vi "Calculate_Tolerance.vi"(2 "error in (no error)":errorcluster, 3 "State":T1=enum."Wait for something", 4 "Data":T2 {"Shaft"."dmin" format="%#_7g"; "Shaft"."dmax" format="%#_7g"; "Shaft"."Fundamental Dev" format="%#_7g"; "Shaft"."Tolerance Grade (IT) Shaft" format="%#_7g"; "Hole"."Dmin" format="%#_7g"; "Hole"."Tolerance Grade (IT)" format="%#_7g"}) -> (0 "error out":errorcluster, 1 "State":T1=enum."Wait for something")   [LabVIEW 2023]
uses:
  TypeDef/Data_Cluster.ctl
  <vilib>/MGI/Panel Manager/Panel/Panel/Window/Window.lvclass
  TypeDef/Units.ctl
  TypeDef/Method_Info.ctl
  TypeDef/Hole_Data.ctl
  TypeDef/Shaft_Data.ctl
  TypeDef/State.ctl
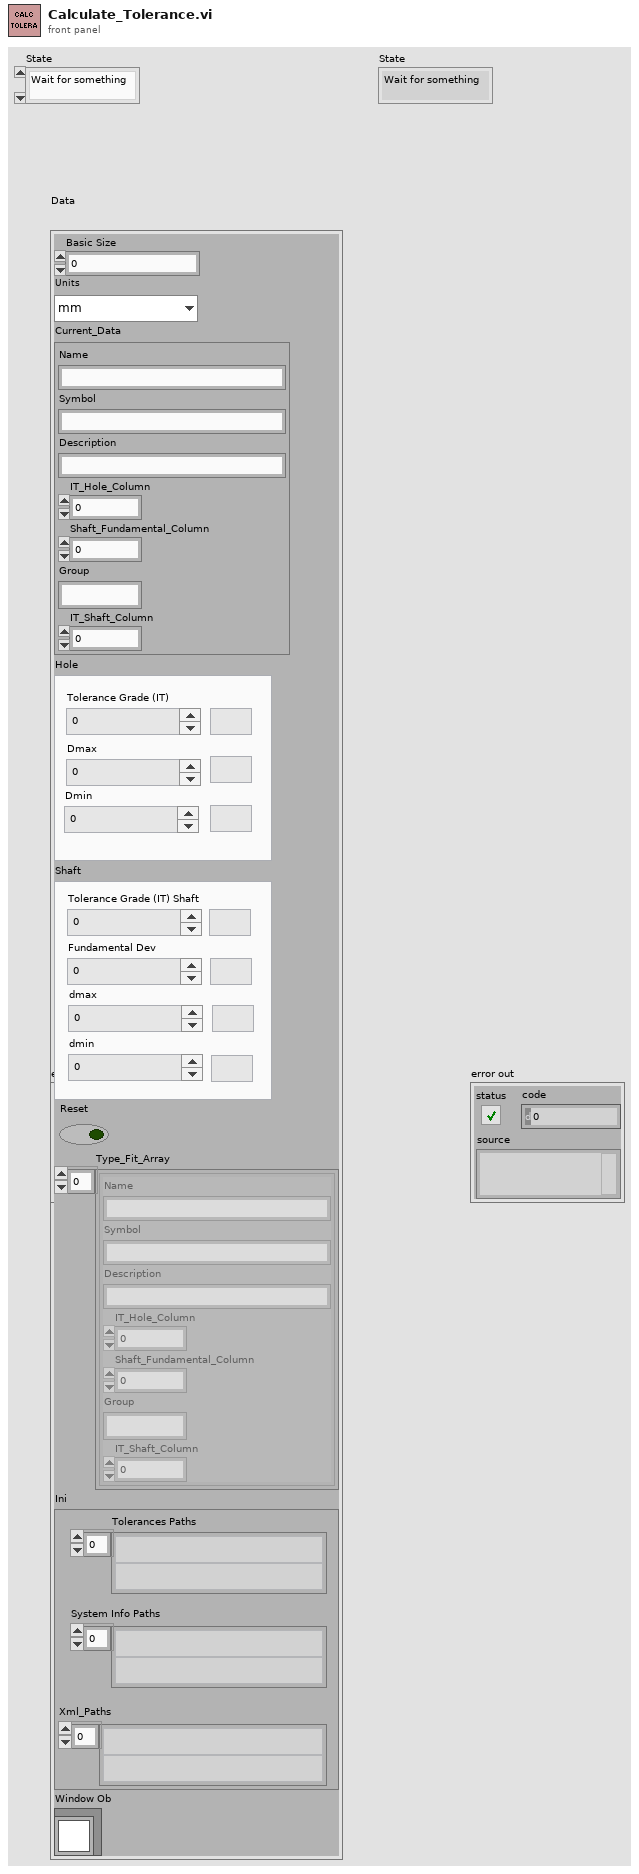
[diagram p1: front panel]
types:
  T1 = typedef "State.ctl" = enum16{"Initialize", "Wait for something", "Method_Description", "Tolerance Grade Hole", "Dmax-min", "Shaft Fudamental", "Shaft Tolerance Grade", "dmax-dmin", "Display Values"}
  T2 = typedef "Data_Cluster.ctl" = cluster{"Basic Size ":dbl, "Units":T3, "Current_Data":T4, "Hole":T5, "Shaft":T6, "Reset":bool, "Type_Fit_Array":T4[], "Ini":cluster{"Tolerances Paths":path[], "System Info Paths":path[], "Xml_Paths":path[]}, "Window Ob":refnum<class "Window.lvclass">}
  T3 = typedef "Units.ctl" = enum16{"mm", "in"}
  T4 = typedef "Method_Info.ctl" = cluster{"Name":string, "Symbol":string, "Description":string, "IT_Hole_Column":i32, "Shaft_Fundamental_Column":i32, "Group":string, "IT_Shaft_Column":i32}
  T5 = typedef "Hole_Data.ctl" = cluster{"Tolerance Grade (IT)":dbl, "Dmax":dbl, "Units Hole":cluster{"units_it":string, "units_Dmax\nUnits_Dmax":string, "Units_Dmin":string}, "Dmin":dbl}
  T6 = typedef "Shaft_Data.ctl" = cluster{"Tolerance Grade (IT) Shaft":dbl, "Units Shaft":cluster{"Units_FundamentalDev":string, "Units_dmax":string, "Units_dmin":string, "Units_IT_Shaft":string}, "Fundamental Dev":dbl, "dmax":dbl, "dmin":dbl}
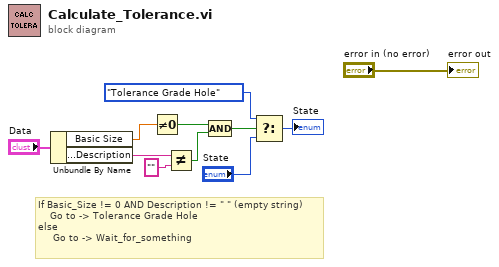
[diagram p0: block diagram]
diagram:
  # "If Basic_Size != 0 AND Description != \" \" (empty string)\n    Go to -> Tolerance Grade Hole\nelse \n     Go to -> Wait_for_something"
  n1 = Unbundle By Name("Data") -> ("Basic Size"=w9:dbl, "Current_Data.Description"=w5:string)
  n2 = Not Equal To 0?(x=w9) -> (x != 0?=w6:bool)
  n3 = Not Equal?(x=w5, y="" ("Data.Method")) -> (x != y?=w3:bool)
  n4 = Compound Arithmetic op=AND(w6, w3) -> (w11:bool)
  n5 = Select(t=State."Tolerance Grade Hole", s=w11, f="State") -> (s? t:f=→"State":T1)
  "error out" <- "error in (no error)"
